vi "DFConfig XPointers to String.vi"(3 "XPointers (empty)":string[](array[string])) -> (1 "xpointer":string)   [LabVIEW 2011]
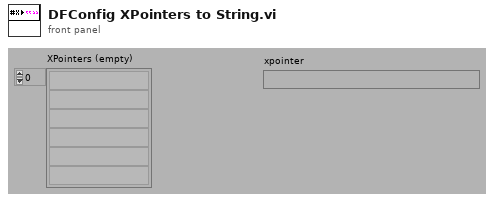
[diagram p1: front panel]
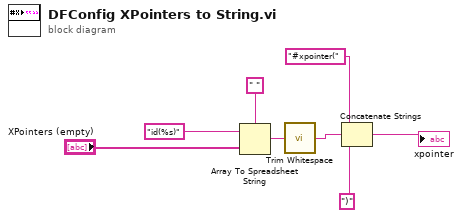
[diagram p0: block diagram]
diagram:
  n1 = Array To Spreadsheet String(delimiter (Tab)=" " ("Tag (\"\")"), array="XPointers (empty)", 3:"id(%s)" ("Tag (\"\")")) -> (spreadsheet string=w2:string)
  n2 = call <vilib>:"Trim Whitespace.vi"("string"=w2) -> ("trimmed string"=w1:string)  [unwired: 1 in]
  n3 = Concatenate Strings("#xpointer(" ("Tag (\"\")"), w1, ")" ("Tag (\"\")")) -> (→"xpointer":string)
